vi "Instrument Manager Loop.vi"(8 "System Control":refnum<queue>, 11 "Optimizer Manager":refnum<queue>) -> (0 "error out":errorcluster)   [LabVIEW 2020, in "Deep Reaction Optimizer Control Panel.lvlib" / "Instrument Manager.lvlib"]
uses:
  Instrument Manager/Instrument Manager.lvlib
  support/Message Queue/Message Cluster.ctl
  Instrument Manager/Instrument State.ctl
  <vilib>/addons/zeromq/zmq_context.lvclass
  <vilib>/addons/zeromq/zmq_socket.lvclass
  <vilib>/addons/zeromq/socket_type.ctl
  <vilib>/addons/zeromq/poll_type.ctl
  <vilib>/Utility/error.llb/Error Cluster From Error Code.vi
  <vilib>/addons/zeromq/zmq_poll_scalar.vi
  <vilib>/ErrorRing/Error Ring.xnode
  support/Message Queue/Message Queue.lvlib
  Deep Reaction Optimizer Control Panel.lvlib
  <vilib>/addons/zeromq/zeromq.lvlib
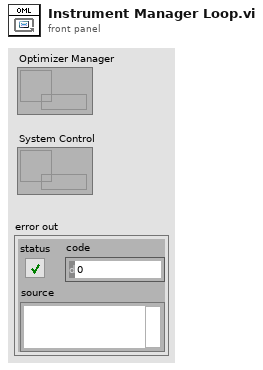
[diagram p1: front panel]
types:
  T1 = typedef "zeromq.lvlib/socket_type.ctl" = enum8{"ZMQ_PAIR", "ZMQ_PUB", "ZMQ_SUB", "ZMQ_REQ", "ZMQ_REP", "ZMQ_DEALER", "ZMQ_ROUTER", "ZMQ_PULL", "ZMQ_PUSH", "ZMQ_XPUB", "ZMQ_XSUB"}
  T2 = typedef "Deep Reaction Optimizer Control Panel.lvlib/Instrument Manager.lvlib/Instrument State.ctl" = cluster{"Context":refnum<class "zmq_context.lvclass">, "Socket":refnum<class "zmq_socket.lvclass">, "Running Since":timestamp, "New Parameters (values)":cluster{"Time Stamp":timestamp, "Name":string[], "Value":dbl[]}, "Optimizer Path":path, "Running":bool, "Response Counter":u8, "Response Timeout (ms)":u32, "Response Retries":u32, "Endpoint":string, "Starting up?":bool, "New Parameters (percents)":cluster{"Time Stamp":timestamp, "Name":string[], "Value":dbl[]}, "Flow Rate Constant":dbl, "Yield":dbl}
  T3 = typedef "zeromq.lvlib/poll_type.ctl" = enum16{"None", "In", "Out", "In/Out"}
  T4 = cluster{"seconds since 1Jan1904":timestamp, string[], dbl[]}
  T5 = cluster{"Time Stamp":timestamp, "Name":string[], "Value":dbl[]}
  T6 = typedef "zeromq.lvlib/error_type.ctl" = enum16{"No Error", "EUNKNOWN", "ENOTSUP", "EPROTONOSUPPORT", "ENOBUFS", "ENETDOWN", "EADDRINUSE", "EADDRNOTAVAIL", "ECONNREFUSED", "EINPROGRESS", "ENOTSOCK", "EMSGSIZE", "EAFNOSUPPORT", "ENETUNREACH", "ECONNABORT", "ECONNRESET", "ENOTCONN", "ETIMEDOUT", "EHOSTUNREACH", "ENETRESET", "EBUSY", "EINVAL", "ENODEV", "EFAULT", "EINTR", "ENOENT", "ENOMEM", "EAGAIN", "EMFILE", "EFSM", "ENOCOMPATPROTO", "ETERM", "EMTHREAD", "Invalid"}
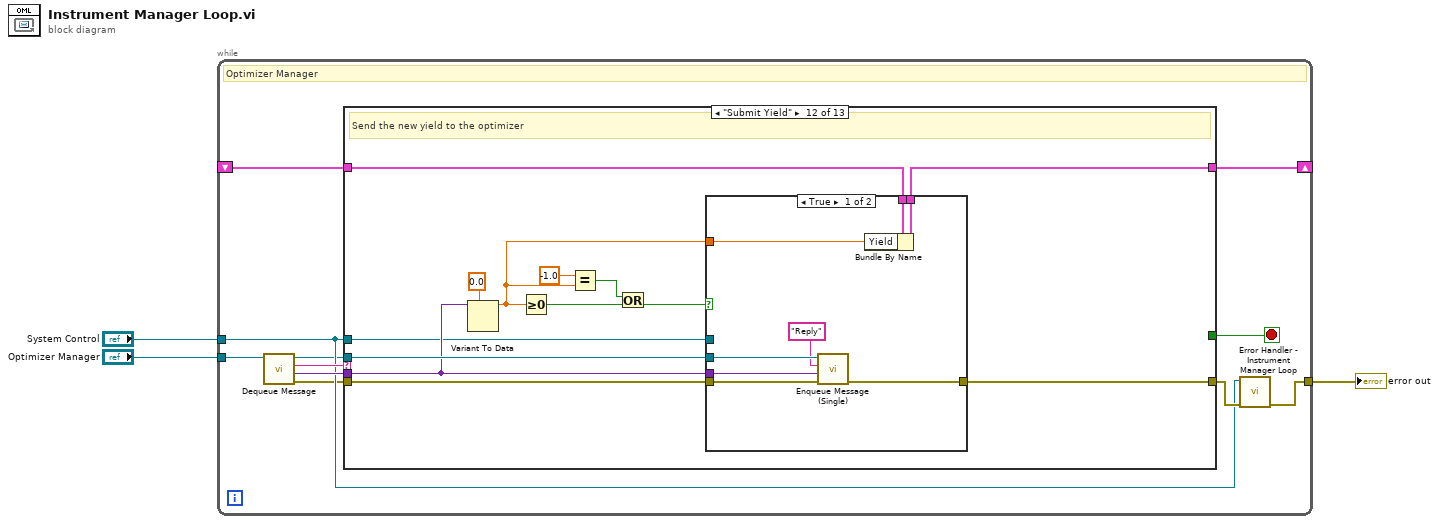
[diagram p0: block diagram]
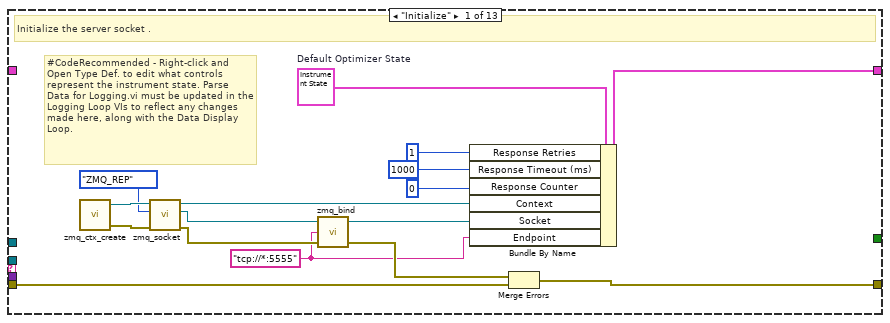
[diagram p2: hidden frame]
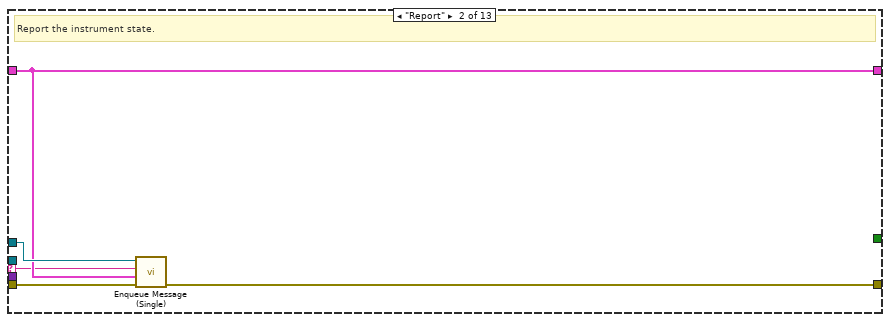
[diagram p3: hidden frame]
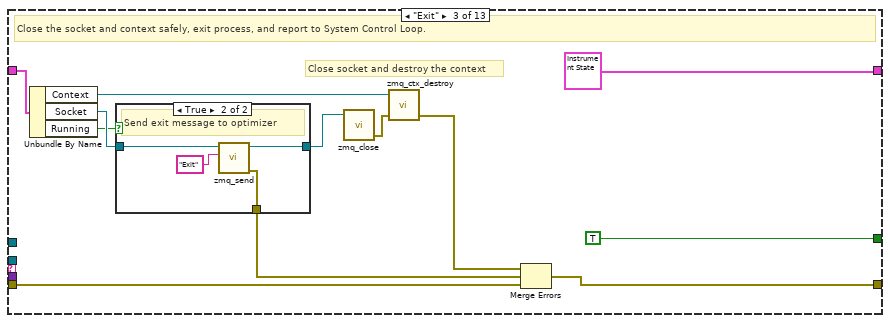
[diagram p4: hidden frame]
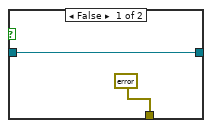
[diagram p5: hidden frame]
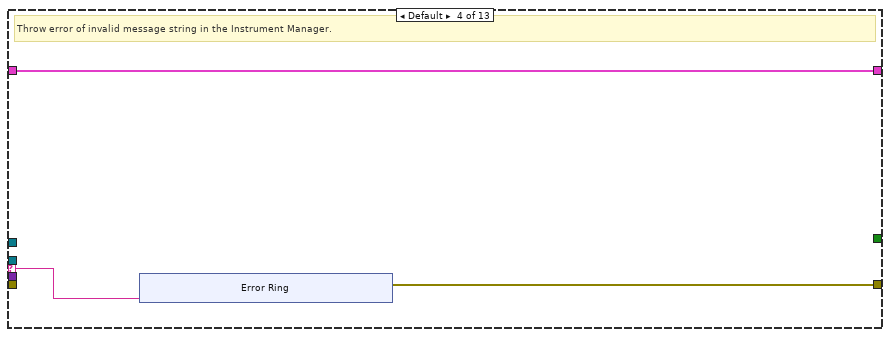
[diagram p6: hidden frame]
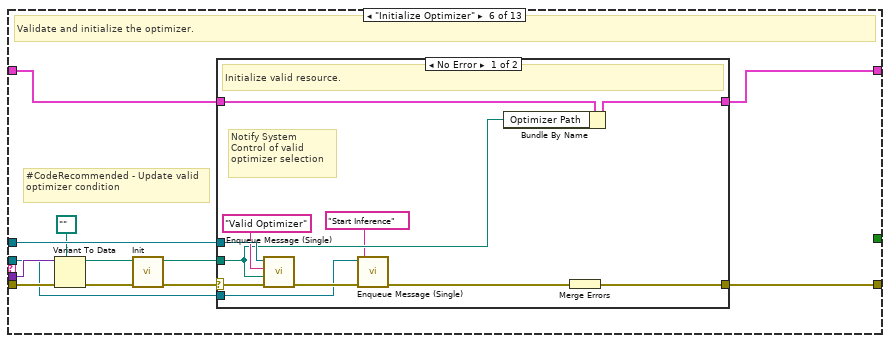
[diagram p8: hidden frame]
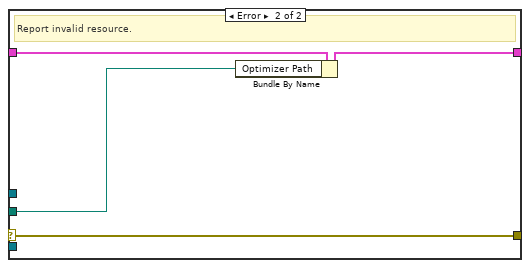
[diagram p9: hidden frame]
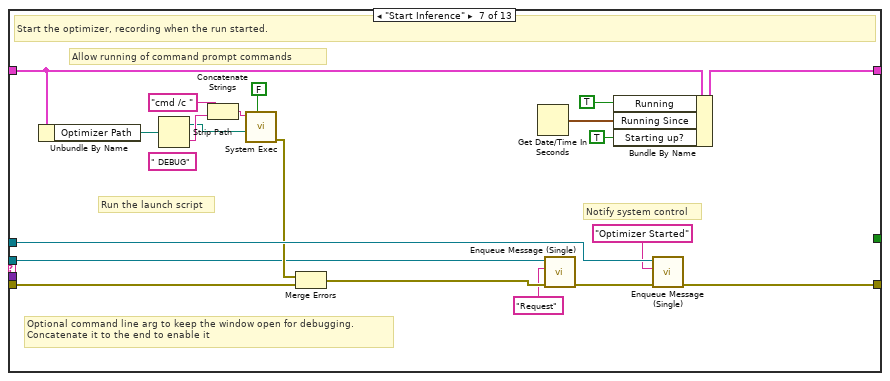
[diagram p10: hidden frame]
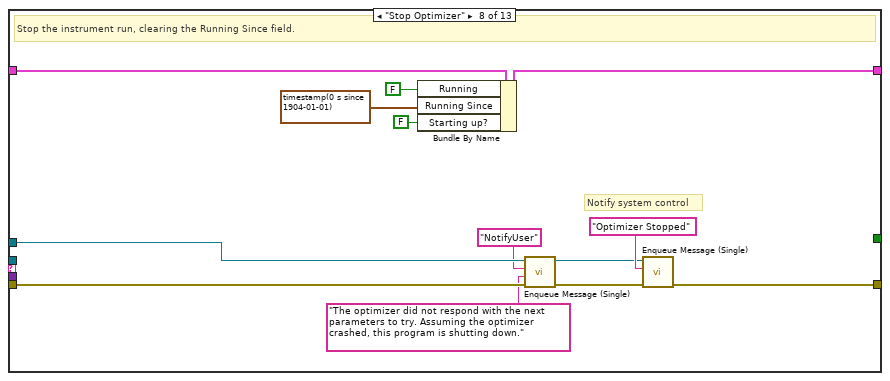
[diagram p11: hidden frame]
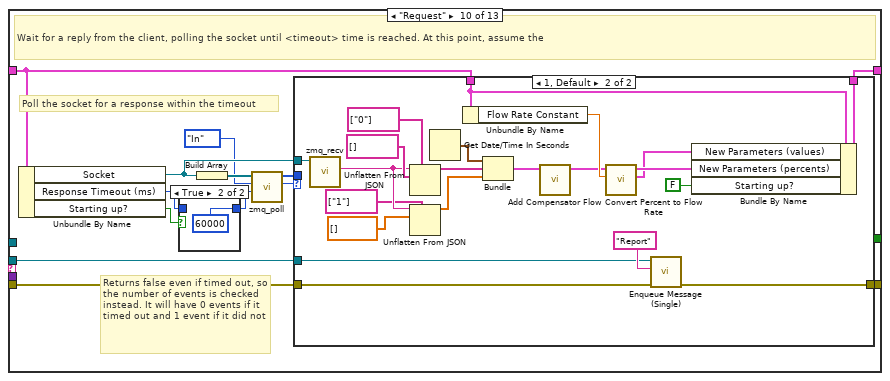
[diagram p13: hidden frame]
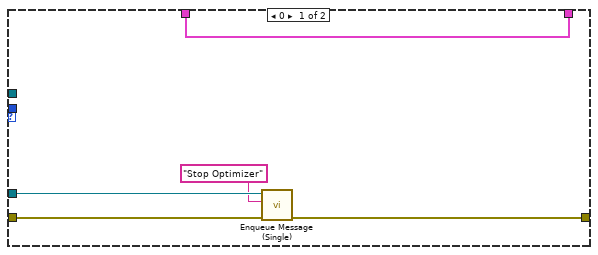
[diagram p15: hidden frame]
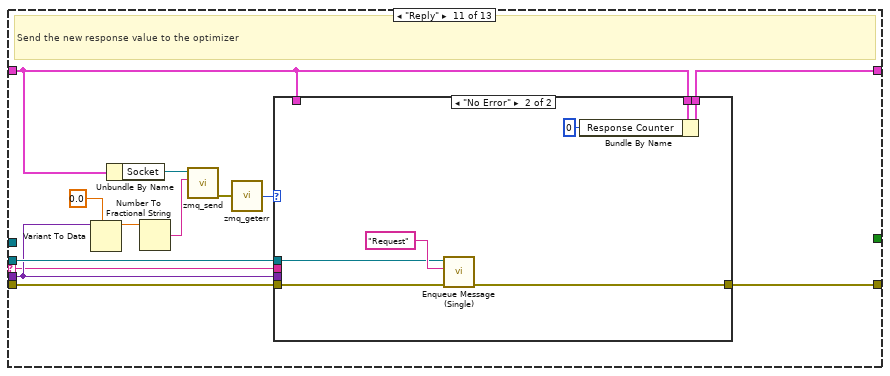
[diagram p16: hidden frame]
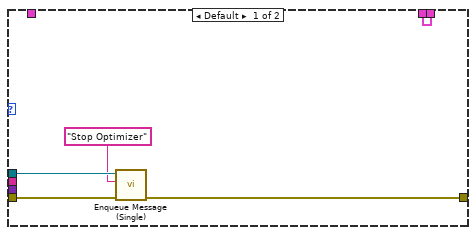
[diagram p17: hidden frame]
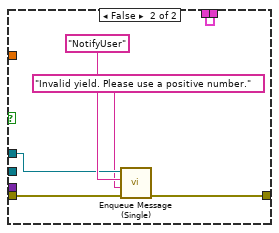
[diagram p18: hidden frame]
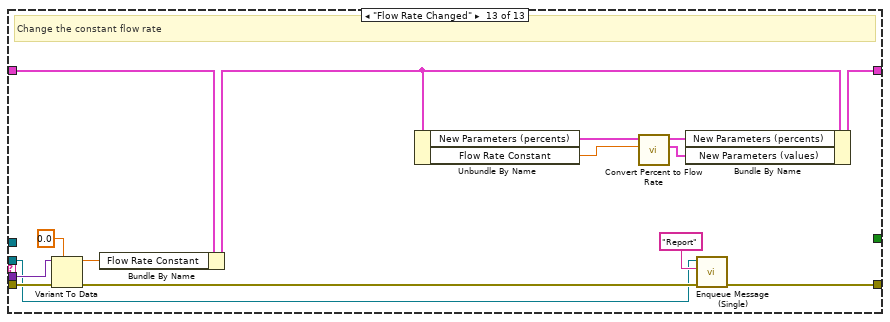
[diagram p19: hidden frame]
diagram:
  n1 = while {
    tunnel: "Optimizer Manager" -> [w14]
    tunnel: "System Control" -> [w6]
    tunnel: [w10] -> w1
    shift-right: [w8] -> _
    shift-left: _ -> [w9]
    stop <- w7 stop-if-true
    # "Optimizer Manager"
    n2 = call "Dequeue Message.vi"("Message Queue"=w14) -> ("error out"=w5:errorcluster, "Message Data"=w12:variant, "Message"=w13:string, "dup Message Queue"=w4:refnum<queue>)  [unwired: 7 in]
    n3 = case shown="\"Submit Yield\"" w13 {
      selector: w13 -> [_ w31 _ w55 _ _ _ _ _ _ w170 _ _]
      tunnel: w4 -> [_ _ _ _ _ w66 w95 _ _ w134 w175 w206 w226]
      tunnel: w6 -> [_ w34 _ _ _ w68 w110 w117 _ _ _ w200 _]
      tunnel: w12 -> [_ _ _ _ _ w74 _ _ _ _ w171 w203 w233]
      tunnel: w5 -> [w30 w35 w42 _ w64 w73 w112 w118 w127 w133 w174 w205 w234]
      tunnel: [w24 w33 w45 w54 w64 w77 w111 w124 w127 w135 w169 w204 w228] -> w11
      tunnel: w9 -> [_ w32 w41 w56 w65 w76 w105 w125 w126 w139 w173 w195 w235]
      tunnel: [w27 w32 T2 {"Context"=refnum, "Socket"=refnum, "Running Since"=timestamp(0 s since 1904-01-01), "New Parameters (values)"={"Time Stamp"=timestamp(0 s since 1904-01-01), "Name"=[], "Value"=[]}, "Optimizer Path"=path "", "Running"=FALSE, "Response Counter"=0, "Response Timeout (ms)"=0, "Response Retries"=0, "Endpoint"="", "Starting up?"=FALSE, "New Parameters (percents)"={"Time Stamp"=timestamp(0 s since 1904-01-01), "Name"=[], "Value"=[]}, "Flow Rate Constant"=0.0, "Yield"=0.0} w56 w65 w75 w108 w122 w126 w140 w172 w194 w224] -> w8
      tunnel: [_ _ TRUE _ _ _ _ _ _ _ _ _ _] -> w7
      frame "Initialize" {
        w15 = "tcp://*:5555" ("endpoint")
        w28 = T2 {"Context"=refnum, "Socket"=refnum, "Running Since"=timestamp(0 s since 1904-01-01), "New Parameters (values)"={"Time Stamp"=timestamp(0 s since 1904-01-01), "Name"=[], "Value"=[]}, "Optimizer Path"=path "", "Running"=FALSE, "Response Counter"=0, "Response Timeout (ms)"=0, "Response Retries"=0, "Endpoint"="", "Starting up?"=FALSE, "New Parameters (percents)"={"Time Stamp"=timestamp(0 s since 1904-01-01), "Name"=[], "Value"=[]}, "Flow Rate Constant"=0.0, "Yield"=0.0}  # Default Optimizer State
        # "#CodeRecommended - Right-click and Open Type Def. to edit what controls represent the instrument state. Parse Data for Logging.vi must be updated in the Logging Loop VIs to reflect any changes made here, along with the Data Display Loop."
        # "Initialize the server socket ."
        n4 = call <vilib>:"zmq_ctx_create.vi"() -> ("error out"=w29:errorcluster, "context out"=w26:refnum<class "zmq_context.lvclass">)  [unwired: 4 in]
        n5 = call <vilib>:"zmq_socket.vi"("error in"=w29, "socket type"=socket_type."ZMQ_REP", "context in"=w26) -> ("error out"=w18:errorcluster, "socket out"=w17:refnum<class "zmq_socket.lvclass">, "context out"=w25:refnum<class "zmq_context.lvclass">)  [unwired: 2 in]
        n6 = call <vilib>:"zmq_bind.vi"("error in"=w18, "endpoint"=w15, "socket in"=w17) -> ("error out"=w19:errorcluster, "socket out"=w20:refnum<class "zmq_socket.lvclass">)  [unwired: 1 in]
        n7 = Bundle By Name(cluster=w28, "Response Retries"=u32 1 ("Consecutive Timeouts Before Heartbeat"), "Response Timeout (ms)"=u32 1000 ("Timeout (ms)"), "Response Counter"=u8 0 ("Consecutive Timeouts"), "Context"=w25, "Socket"=w20, "Endpoint"=w15) -> (w27:T2)
        n8 = Merge Errors(w19, w30) -> (w24:errorcluster)
      }
      frame "Report" {
        # "Report the instrument state."
        n9 = call "Enqueue Message (Single).vi"("error in (no error)"=w35, "Message Data"=w32, "Message"=w31, "Message Queue"=w34) -> ("error out"=w33:errorcluster)  [unwired: 6 in, 1 out]
      }
      frame "Exit" {
        # "Close socket and destroy the context"
        # "Close the socket and context safely, exit process, and report to System Control Loop."
        n10 = Unbundle By Name(w41) -> ("Context"=w43:refnum<class "zmq_context.lvclass">, "Socket"=w40:refnum<class "zmq_socket.lvclass">, "Running"=w36:bool)
        n11 = case shown="True" w36 {
          tunnel: w40 -> [w48 w52]
          tunnel: [w48 w51] -> w39
          tunnel: [errorcluster {"status"=FALSE, "code"=0, "source"=""} ("error out") w50] -> w37
          frame False {
          }
          frame True {
            # "Send exit message to optimizer"
            n12 = call <vilib>:"zmq_send.vi"("data"="Exit", "socket in"=w52) -> ("error out"=w50:errorcluster, "socket out"=w51:refnum<class "zmq_socket.lvclass">)  [unwired: 5 in]
          }
        }
        n13 = call <vilib>:"zmq_close.vi"("socket"=w39) -> ("error out"=w44:errorcluster)  [unwired: 4 in]
        n14 = call <vilib>:"zmq_ctx_destroy.vi"("error in"=w44, "context in"=w43) -> ("error out"=w38:errorcluster)  [unwired: 3 in]
        n15 = Merge Errors(w38, w37, w42) -> (w45:errorcluster)
      }
      frame Default {
        # "Throw error of invalid message string in the Instrument Manager."
        n16 = xnode "Error Ring"("parameter 0"=w55) -> ("error out"=w54:errorcluster)
      }
      frame "--- Copy This Frame ---" {
        # "Copy this frame and add responses to instrument specific messages."
      }
      frame "Initialize Optimizer" {
        # "#CodeRecommended - Update valid optimizer condition"
        # "Validate and initialize the optimizer."
        n17 = Variant To Data(error in=w73, type=path "", Variant=w74) -> (data=w71:path, error out=w72:errorcluster)
        n18 = call "Init.vi"("error in (no error)"=w72, "optimizer path"=w71) -> ("error out"=w69:errorcluster, "optimizer path (out)"=w70:path)  [unwired: 8 in]
        n19 = case shown="No Error" w69 {
          selector: w69 -> [w87 w89]
          tunnel: w70 -> [w83 w90]
          tunnel: [w82 w89] -> w77
          tunnel: w76 -> [w88 w92]
          tunnel: [w84 w91] -> w75
          tunnel: w68 -> [w86 _]
          tunnel: w66 -> [w79 _]
          frame No Error {
            # "Notify System Control of valid optimizer selection"
            # "Initialize valid resource."
            n20 = call "Enqueue Message (Single).vi"("error in (no error)"=w87, "Message Data"=w83, "Message"="Valid Optimizer", "Message Queue"=w86) -> ("error out"=w81:errorcluster)  [unwired: 6 in, 1 out]
            n21 = call "Enqueue Message (Single).vi"("error in (no error)"=w81, "Message"="Start Inference", "Message Queue"=w79) -> ("error out"=w80:errorcluster)  [unwired: 7 in, 1 out]
            n22 = Bundle By Name(cluster=w88, "Optimizer Path"=w83) -> (w84:T2)
            n23 = Merge Errors(w80) -> (w82:errorcluster)
          }
          frame Error {
            # "Report invalid resource."
            n24 = Bundle By Name(cluster=w92, "Optimizer Path"=w90) -> (w91:T2)
          }
        }
      }
      frame "Start Inference" {
        (unwired) " DEBUG" ("string")
        # "Optional command line arg to keep the window open for debugging.\nConcatenate it to the end to enable it"
        # "Allow running of command prompt commands"
        # "Run the launch script"
        # "Notify system control"
        # "Start the optimizer, recording when the run started."
        n25 = Unbundle By Name(w105) -> ("Optimizer Path"=w102:path)
        n26 = Strip Path(path=w102) -> (stripped path=w100:path, name=w101:string)
        n27 = Concatenate Strings("cmd /c " ("string"), w101) -> (w99:string)
        n28 = call <vilib>:"System Exec.vi"("wait until completion? (T)"=FALSE, "working directory"=w100, "command line"=w99) -> ("error out"=w103:errorcluster)  [unwired: 5 in, 3 out]
        n29 = Merge Errors(w103, w112) -> (w96:errorcluster)
        n30 = Get Date/Time In Seconds() -> (seconds since 1Jan1904=w106:timestamp)
        n31 = call "Enqueue Message (Single).vi"("error in (no error)"=w96, "Message"="Request", "Message Queue"=w95) -> ("error out"=w97:errorcluster)  [unwired: 7 in, 1 out]
        n32 = Bundle By Name(cluster=w105, "Running"=TRUE, "Running Since"=w106, "Starting up?"=TRUE) -> (w108:T2)
        n33 = call "Enqueue Message (Single).vi"("error in (no error)"=w97, "Message"="Optimizer Started", "Message Queue"=w110) -> ("error out"=w111:errorcluster)  [unwired: 7 in, 1 out]
      }
      frame "Stop Optimizer" {
        # "Notify system control"
        # "Stop the instrument run, clearing the Running Since field."
        n34 = Bundle By Name(cluster=w125, "Running"=FALSE, "Running Since"=timestamp(0 s since 1904-01-01), "Starting up?"=FALSE) -> (w122:T2)
        n35 = call "Enqueue Message (Single).vi"("error in (no error)"=w118, "Message Data"="The optimizer did not respond with the next parameters to try. Assuming the optimizer crashed, this program is shutting down.", "Message"="NotifyUser", "Message Queue"=w117) -> ("error out"=w119:errorcluster, "dup Message Queue"=w116:refnum<queue>)  [unwired: 6 in]
        n36 = call "Enqueue Message (Single).vi"("error in (no error)"=w119, "Message"="Optimizer Stopped", "Message Queue"=w116) -> ("error out"=w124:errorcluster)  [unwired: 7 in, 1 out]
      }
      frame "--- Copy for Get State Messages ---" {
        # "#CodeNeeded - Use the Bundle by Name function to bundle the new state value into the Instrument State cluster."
        # "#CodeNeeded - Add instrument driver call to query the instrument state requested"
        # "Duplicate this case for messages cases that will query the instrument state."
      }
      frame "Request" {
        # "Returns false even if timed out, so the number of events is checked instead. It will have 0 events if it timed out and 1 event if it did not"
        # "Poll the socket for a response within the timeout"
        # "Wait for a reply from the client, polling the socket until <timeout> time is reached. At this point, assume the"
        n37 = Unbundle By Name(w139) -> ("Socket"=w137:refnum<class "zmq_socket.lvclass">, "Response Timeout (ms)"=w129:u32, "Starting up?"=w130:bool)
        n38 = case shown="True" w130 {
          tunnel: w129 -> [w141 _]
          tunnel: [w141 u32 60000 ("Response Timeout (ms)")] -> w128
          frame False {
          }
          frame True {
          }
        }
        n39 = Build Array(w137) -> (w138:refnum<class "zmq_socket.lvclass">[])
        n40 = call-poly <vilib>:"zmq_poll.vi"("timeout"=w128, "poll type"=poll_type."In", "sockets"=w138) -> ("nevents"=w131:i32, "polled events"=w132:T3[])  [unwired: 1 in, 2 out]
        n41 = case shown="1, Default" w131 {
          tunnel: [w147 w168] -> w140
          tunnel: w139 -> [w147 w152]
          tunnel: w137 -> [_ w167]
          tunnel: w133 -> [w146 w166]
          tunnel: [w143 w164] -> w135
          tunnel: w134 -> [w145 w163]
          tunnel: w132 -> [_ _]
          frame 0 {
            n42 = call "Enqueue Message (Single).vi"("error in (no error)"=w146, "Message"="Stop Optimizer", "Message Queue"=w145) -> ("error out"=w143:errorcluster)  [unwired: 7 in, 1 out]
          }
          frame 1, Default {
            n43 = call <vilib>:"zmq_recv.vi"("socket in"=w167) -> ("data"=w160:string)  [unwired: 4 in, 4 out]
            n44 = Unflatten From JSON(path=string[] ["0"], JSON string=w160, type and defaults=string[] []) -> (value=w155:string[])  [unwired: 4 in, 1 out]
            n45 = Unflatten From JSON(path=string[] ["1"], JSON string=w160, type and defaults=dbl[] []) -> (value=w154:dbl[])  [unwired: 4 in, 1 out]
            n46 = Get Date/Time In Seconds() -> (seconds since 1Jan1904=w156:timestamp)
            n47 = Unbundle By Name(w152) -> ("Flow Rate Constant"=w151:dbl)
            n48 = Bundle("seconds since 1Jan1904"=w156, w155, w154) -> (w153:T4)  [unwired: 1 in]
            n49 = call "Add Compensator Flow.vi"("New Parameters (percents)"=w153) -> ("New Parameters (percents) out"=w148:T5)  [unwired: 9 in, 1 out]
            n50 = call "Convert Percent to Flow Rate.vi"("Flow Rate Constant"=w151, "New Parameters (percents)"=w148) -> ("New Parameters (values) out"=w149:T5, "New Parameters (percents) out"=w150:T5)  [unwired: 8 in]
            n51 = call "Enqueue Message (Single).vi"("error in (no error)"=w166, "Message"="Report", "Message Queue"=w163) -> ("error out"=w164:errorcluster)  [unwired: 7 in, 1 out]
            n52 = Bundle By Name(cluster=w152, "New Parameters (values)"=w149, "New Parameters (percents)"=w150, "Starting up?"=FALSE) -> (w168:T2)
          }
        }
      }
      frame "Reply" {
        # "Send the new response value to the optimizer"
        n53 = Variant To Data(type=0.0, Variant=w171) -> (data=w179:dbl)  [unwired: 1 in, 1 out]
        n54 = Unbundle By Name(w173) -> ("Socket"=w181:refnum<class "zmq_socket.lvclass">)
        n55 = Number To Fractional String(number=w179) -> (F-format string=w178:string)  [unwired: 3 in]
        n56 = call <vilib>:"zmq_send.vi"("data"=w178, "socket in"=w181) -> ("error out"=w177:errorcluster)  [unwired: 5 in, 1 out]
        n57 = call <vilib>:"zmq_geterr.vi"("error in"=w177) -> ("type"=w176:T6)
        n58 = case shown="\"No Error\"" w176 {
          tunnel: w174 -> [w185 w191]
          tunnel: w175 -> [w186 w192]
          tunnel: w170 -> [_ _]
          tunnel: [w184 w190] -> w169
          tunnel: w173 -> [w182 w189]
          tunnel: [w182 w188] -> w172
          tunnel: w173 -> [_ _]
          tunnel: w171 -> [_ _]
          frame Default {
            n59 = call "Enqueue Message (Single).vi"("error in (no error)"=w185, "Message"="Stop Optimizer", "Message Queue"=w186) -> ("error out"=w184:errorcluster)  [unwired: 7 in, 1 out]
          }
          frame "No Error" {
            n60 = call "Enqueue Message (Single).vi"("error in (no error)"=w191, "Message"="Request", "Message Queue"=w192) -> ("error out"=w190:errorcluster)  [unwired: 7 in, 1 out]
            n61 = Bundle By Name(cluster=w189, "Response Counter"=u8 0 ("Timeout Counter")) -> (w188:T2)
          }
        }
      }
      frame "Submit Yield" {
        # "Send the new yield to the optimizer"
        n62 = Variant To Data(type=0.0, Variant=w203) -> (data=w196:dbl)  [unwired: 1 in, 1 out]
        n63 = Greater Or Equal To 0?(x=w196) -> (x >= 0?=w201:bool)
        n64 = Equal?(x=-1.0, y=w196) -> (x = y?=w198:bool)
        n65 = Or(x=w198, y=w201) -> (x .or. y?=w199:bool)
        n66 = case shown="True" w199 {
          tunnel: w206 -> [w214 _]
          tunnel: w205 -> [w213 w220]
          tunnel: [w212 w219] -> w204
          tunnel: w203 -> [w210 _]
          tunnel: w200 -> [_ w217]
          tunnel: w196 -> [w207 _]
          tunnel: w195 -> [w209 w215]
          tunnel: [w208 w215] -> w194
          frame True {
            n67 = call "Enqueue Message (Single).vi"("error in (no error)"=w213, "Message Data"=w210, "Message"="Reply", "Message Queue"=w214) -> ("error out"=w212:errorcluster)  [unwired: 6 in, 1 out]
            n68 = Bundle By Name(cluster=w209, "Yield"=w207) -> (w208:T2)
          }
          frame False {
            n69 = call "Enqueue Message (Single).vi"("error in (no error)"=w220, "Message Data"="Invalid yield. Please use a positive number.", "Message"="NotifyUser", "Message Queue"=w217) -> ("error out"=w219:errorcluster)  [unwired: 6 in, 1 out]
          }
        }
      }
      frame "Flow Rate Changed" {
        # "Change the constant flow rate"
        n70 = Variant To Data(error in=w234, type=0.0, Variant=w233) -> (data=w231:dbl, error out=w229:errorcluster)
        n71 = Bundle By Name(cluster=w235, "Flow Rate Constant"=w231) -> (w223:T2)
        n72 = Unbundle By Name(w223) -> ("New Parameters (percents)"=w222:T5, "Flow Rate Constant"=w225:dbl)
        n73 = call "Convert Percent to Flow Rate.vi"("Flow Rate Constant"=w225, "New Parameters (percents)"=w222) -> ("New Parameters (values) out"=w221:T5, "New Parameters (percents) out"=w230:T5)  [unwired: 8 in]
        n74 = Bundle By Name(cluster=w223, "New Parameters (percents)"=w230, "New Parameters (values)"=w221) -> (w224:T2)
        n75 = call "Enqueue Message (Single).vi"("error in (no error)"=w229, "Message"="Report", "Message Queue"=w226) -> ("error out"=w228:errorcluster)  [unwired: 7 in, 1 out]
      }
    }
    n76 = call "Error Handler - Instrument Manager Loop.vi"("error in (no error)"=w11, "Message Queue"=w6) -> ("dup error in"=w10:errorcluster)  [unwired: 8 in, 1 out]
  }
  "error out" <- w1
